vi "MainControlPane.vi"() -> ()   [LabVIEW 2017]
uses:
  Item.ctl
  Vending State.ctl
  <vilib>/Utility/file.llb/Read Delimited Spreadsheet (string).vi
panel:
  in  "Take Items Button":bool
  in  "Set Angle":dbl
  out "Status":string
  out "Change":dbl
  in  "Insert Money":dbl
  in  "Front Buttons":T1[](array[typedef])
  in  "Motor":bool
  in  "Vending Machine":bool
  # "Vending Machine"
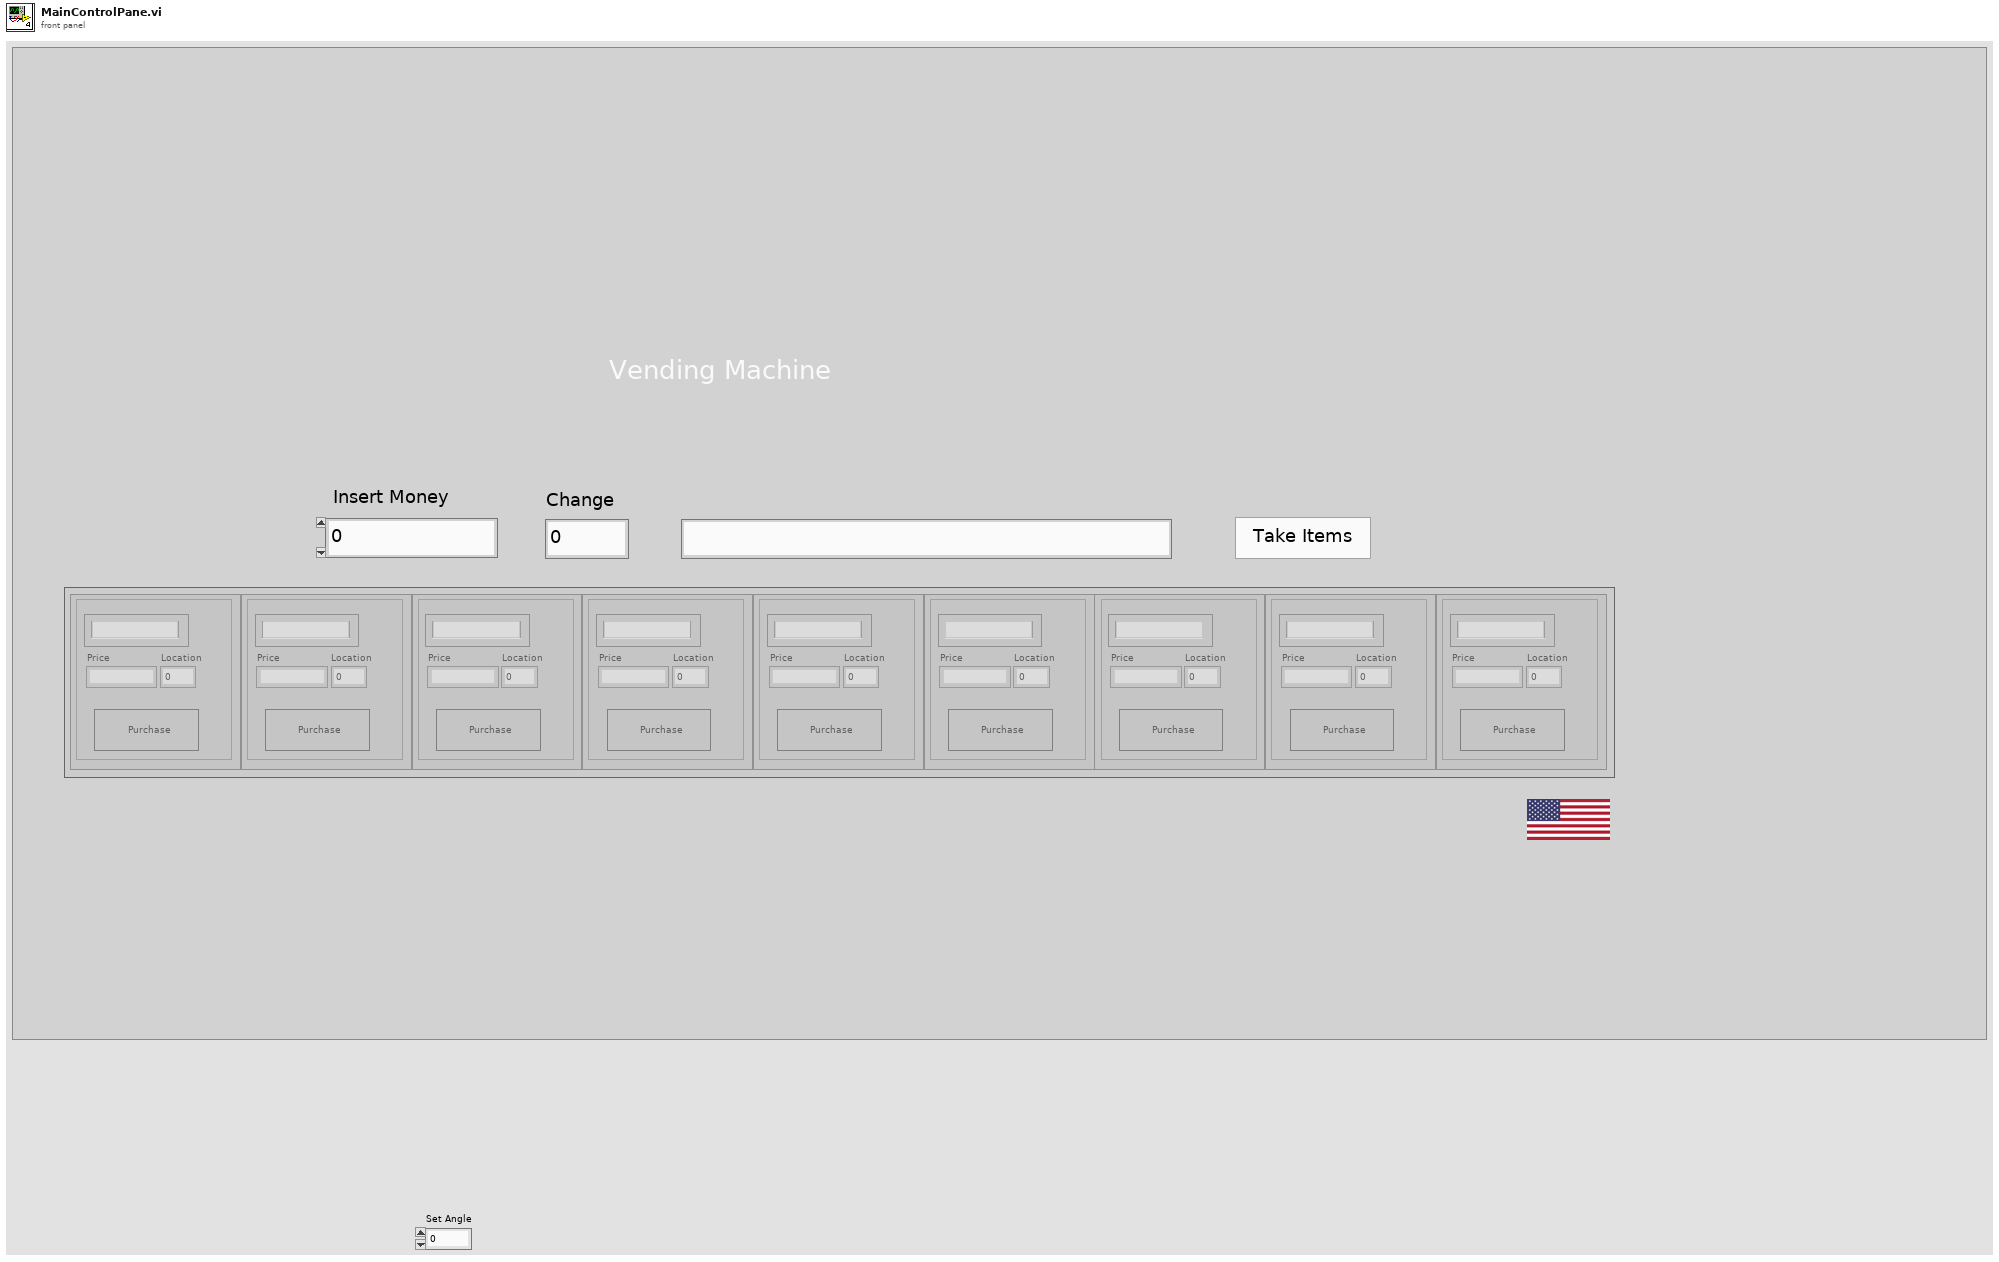
[diagram p1: front panel]
types:
  T1 = typedef "Item.ctl" = cluster{"Button":bool, "Name":string, "Price":string, "Location":dbl}
  T2 = typedef "Vending State.ctl" = enum16{"Wait", "Moving Item", "Reset"}
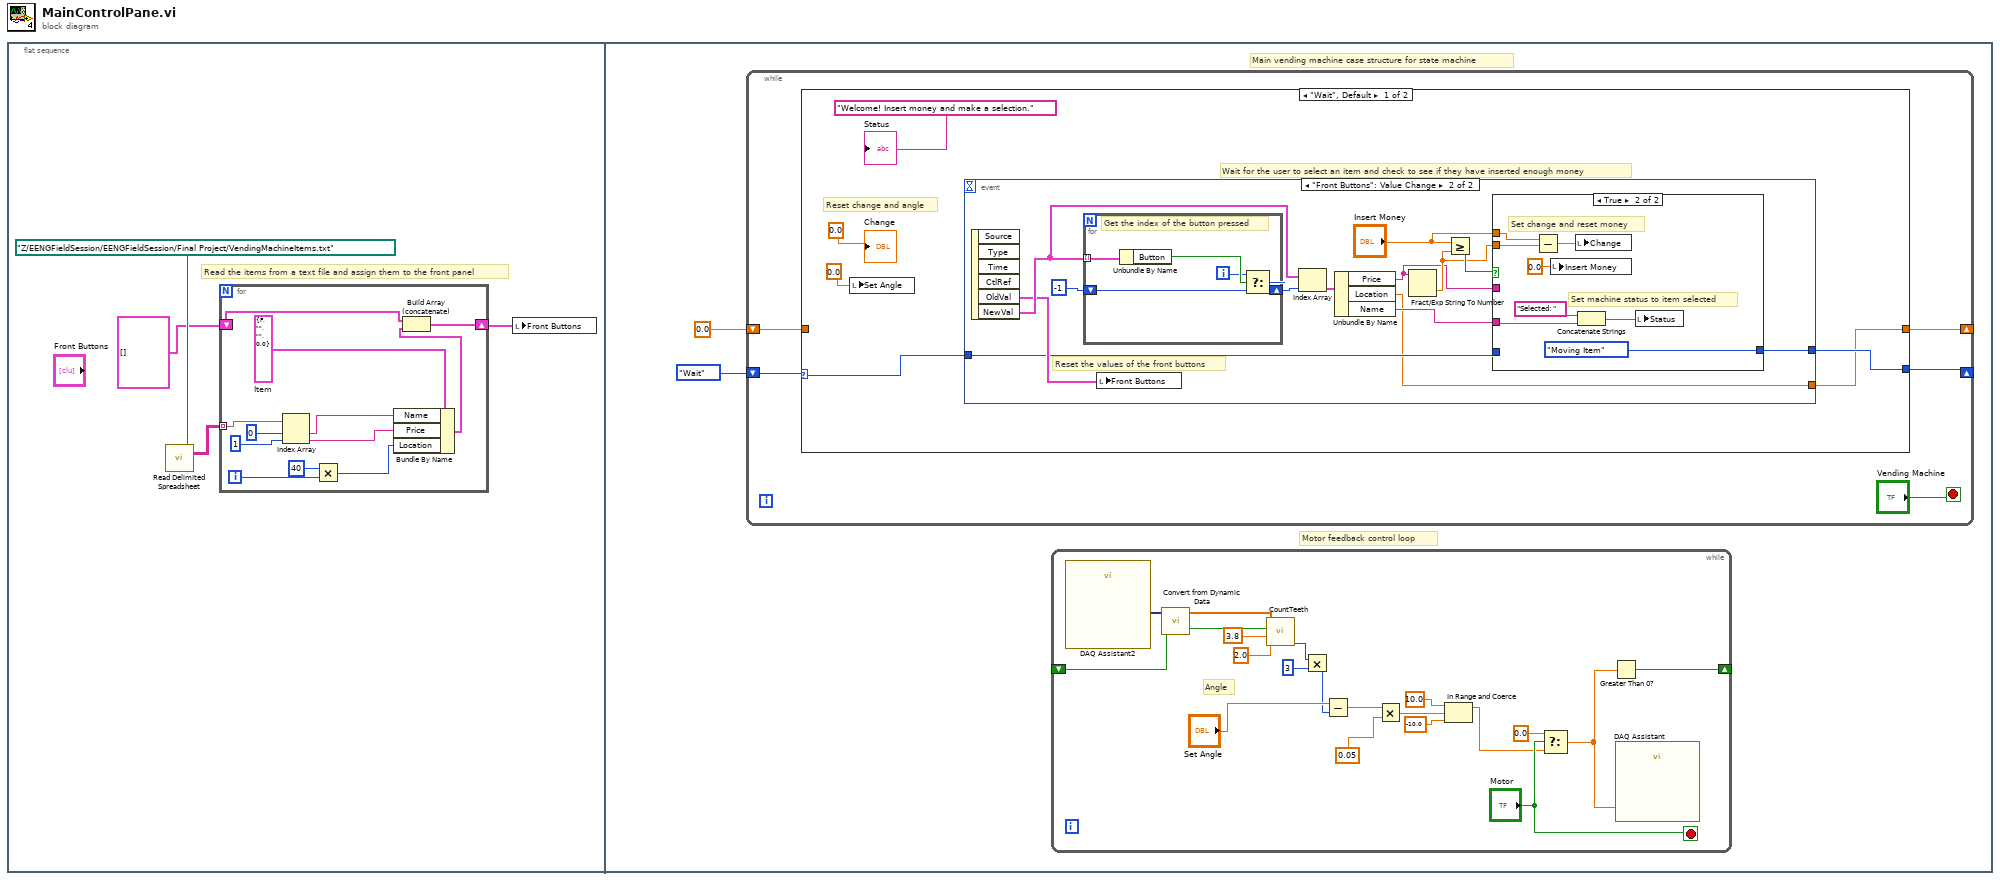
[diagram p0: block diagram]
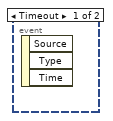
[diagram p2: hidden frame]
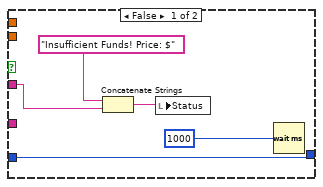
[diagram p3: hidden frame]
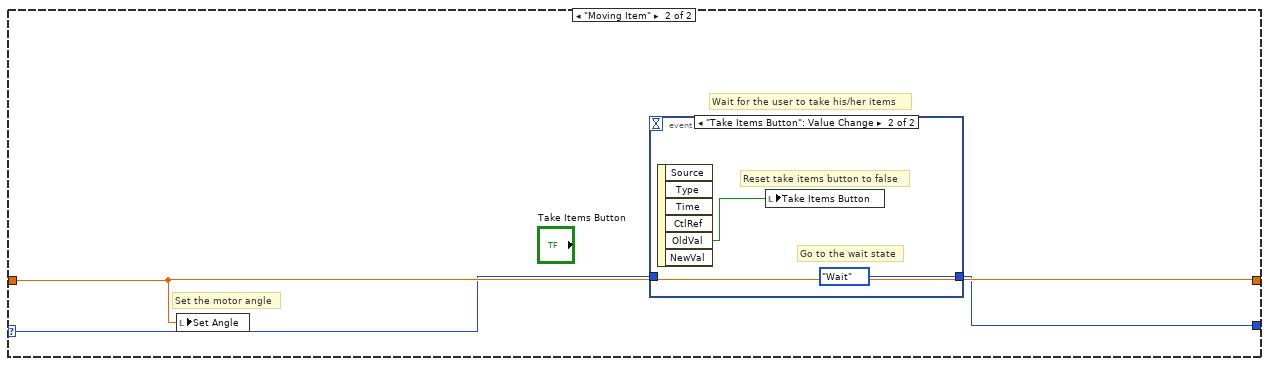
[diagram p4: hidden frame]
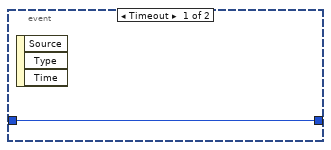
[diagram p5: hidden frame]
diagram:
  n1 = flat-sequence {
    frame #0 {
      # "Read the items from a text file and assign them to the front panel"
      n2 = call-poly <vilib>:"Read Delimited Spreadsheet.vi"("file path (dialog if empty)"=path "Z:/EENGFieldSession/EENGFieldSession/Final Project/VendingMachineItems.txt" ("Path")) -> ("all rows"=w2:string[][])  [unwired: 9 in, 5 out]
      n3 = for {
        tunnel: w2 -> [w16] mode=indexing
        shift-right: [w9] -> w1
        shift-left: T1[] [] ("Array") -> [w10]
        i -> [w7]
        w11 = T1 {"Button"=FALSE, "Name"="", "Price"="", "Location"=0.0}  # Item
        n4 = Index Array(array=w16, index #1=0 ("index"), index #2=1 ("index")) -> (element #1=w13:string, element #2=w12:string)
        n5 = Multiply(x=40, y=w7) -> (x*y=w5:i32)
        n6 = Bundle By Name(cluster=w11, "Name"=w13, "Price"=w12, "Location"=w5) -> (w8:T1)
        n7 = Build Array (concatenate)(w10, w8) -> (w9:T1[])
      }
      n8 = local write "Front Buttons"(w1) -> ()
    }
    frame #1 {
      # "Main vending machine case structure for state machine"
      # "Motor feedback control loop"
      n9 = while {
        shift-right: [w42] -> _
        shift-left: Vending_State."Wait" ("Enum") -> [w41]
        shift-right: [w39] -> _
        shift-left: 0.0 ("Location") -> [w38]
        stop <- "Vending Machine" stop-if-true
        n10 = case shown="\"Wait\", Default" w41 {
          selector: w41 -> [w48 w81]
          tunnel: [w46 w80] -> w42
          tunnel: [w45 w82] -> w39
          tunnel: w38 -> [_ w82]
          frame "Wait", Default {
            # "Reset change and angle"
            # "Wait for the user to select an item and check to see if they have inserted enough money"
            n11 = local write "Set Angle"(0.0 ("Set Angle")) -> ()
            n12 = event shown="[1] \"Front Buttons\": Value Change" {
              selector: _ -> [_ _]
              dyn-events: _ -> [_ _]
              timeout: _ -> [_ _]
              tunnel: w48 -> [_ w51]
              tunnel: [_ w50] -> w46
              tunnel: [_ w49] -> w45
              event Timeout {
                n13 = event-data() -> ()  [unwired: 1 in, 3 out]
              }
              event "Front Buttons": Value Change {
                # "Reset the values of the front buttons"
                n14 = event-data() -> ("OldVal"=w55:T1[], "NewVal"=w59:T1[])  [unwired: 1 in, 4 out]
                n15 = for {
                  tunnel: w59 -> [w79] mode=indexing
                  shift-right: [w75] -> w60
                  shift-left: -1 -> [w76]
                  i -> [w77]
                  # "Get the index of the button pressed"
                  n16 = Unbundle By Name(w79) -> ("Button"=w78:bool)
                  n17 = Select(t=w77, s=w78, f=w76) -> (s? t:f=w75:i32)
                }
                n18 = local write "Front Buttons"(w55) -> ()
                n19 = Index Array(array=w59, index=w60) -> (element=w57:T1)
                n20 = Unbundle By Name(w57) -> ("Price"=w52:string, "Location"=w49:dbl, "Name"=w56:string)
                n21 = Fract/Exp String To Number(string=w52) -> (number=w53:dbl)  [unwired: 3 in, 1 out]
                n22 = Greater Or Equal?(x="Insert Money", y=w53) -> (x >= y?=w58:bool)
                n23 = case shown="True" w58 {
                  tunnel: w56 -> [_ w73]
                  tunnel: "Insert Money" -> [_ w72]
                  tunnel: w53 -> [_ w71]
                  tunnel: w52 -> [w65 _]
                  tunnel: w51 -> [w62 _]
                  tunnel: [w62 Vending_State."Moving Item" ("Enum")] -> w50
                  frame False {
                    n24 = Concatenate Strings("Insufficient Funds! Price: $", w65) -> (w63:string)
                    n25 = local write "Status"(w63) -> ()
                    n26 = Wait (ms)(milliseconds to wait=u32 1000) -> ()  [unwired: 1 out]
                  }
                  frame True {
                    # "Set machine status to item selected"
                    # "Set change and reset money"
                    n27 = Subtract(x=w72, y=w71) -> (x-y=w69:dbl)
                    n28 = local write "Insert Money"(0.0 ("Insert Money")) -> ()
                    n29 = local write "Change"(w69) -> ()
                    n30 = Concatenate Strings("Selected: ", w73) -> (w68:string)
                    n31 = local write "Status"(w68) -> ()
                  }
                }
              }
            }
            "Change" <- 0.0 ("Change")
            "Status" <- "Welcome! Insert money and make a selection." ("Status")
          }
          frame "Moving Item" {
            # "Set the motor angle"
            # "Wait for the user to take his/her items"
            n32 = local write "Set Angle"(w82) -> ()
            n33 = event shown="[1] \"Take Items Button\": Value Change" {
              selector: _ -> [_ _]
              dyn-events: _ -> [_ _]
              timeout: _ -> [_ _]
              tunnel: w81 -> [w83 _]
              tunnel: [w83 Vending_State."Wait" ("Enum")] -> w80
              event Timeout {
                n34 = event-data() -> ()  [unwired: 1 in, 3 out]
              }
              event "Take Items Button": Value Change {
                # "Go to the wait state"
                # "Reset take items button to false"
                n35 = event-data() -> ("OldVal"=w84:bool)  [unwired: 1 in, 5 out]
                n36 = local write "Take Items Button"(w84) -> ()
              }
            }
          }
        }
      }
      n37 = while {
        shift-right: [w29] -> _
        shift-left: _ -> [w28]
        stop <- "Motor" stop-if-true
        # "Angle"
        n38 = call "DAQ Assistant2"() -> ("data"=w37:dynamicdata)  [unwired: 16 in, 3 out]
        n39 = call "Convert from Dynamic Data"("Dynamic Data Type"=w37) -> ("Array"=w27:dbl[])  [unwired: 3 in]
        n40 = call "CountTeeth.vi"("Falling Threshold"=2.0, "Rising Threshold"=3.8, "Direction"=w28, "Array"=w27) -> ("Gear Count"=w26:i32)  [unwired: 7 in]
        n41 = Multiply(x=w26, y=3) -> (x*y=w22:i32)
        n42 = Subtract(x="Set Angle", y=w22) -> (x-y=w20:dbl)
        n43 = Multiply(x=w20, y=0.05) -> (x*y=w35:dbl)
        n44 = In Range and Coerce(upper limit=10.0, x=w35, lower limit=-10.0) -> (coerced(x)=w31:dbl)  [unwired: 1 out]
        n45 = Select(t=0.0, s="Motor", f=w31) -> (s? t:f=w19:dbl)
        n46 = Greater Than 0?(x=w19) -> (x > 0?=w29:bool)
        n47 = call "DAQ Assistant"("data"=w19) -> ()  [unwired: 17 in, 2 out]
      }
    }
  }
